vi "Configure Data Logger.vi"(0 "VISA resource name":refnum<visa-resource-name>, 1 "Data Logging (0: Current)":i32(ring) items=["Current", "Voltage"], 5 "Channel (1)":string="1", 7 "Sample Duration (1 sec)":dbl=1.0, 9 "Sample Interval (0.2 sec)":dbl=0.2, 11 "error in (no error)":errorcluster, 12 "Enable Data Logging (T: Enable)":bool=TRUE, 13 "Enable Extremum (T: Enable)":bool=TRUE) -> (4 "VISA resource name out":refnum<visa-resource-name>, 15 "error out":errorcluster)   [LabVIEW 2020, in "Keysight E36300 Series.lvlib"]
doc: "Configures the data logging.\n\n<b>Note: </b>\nThis VI is only available on the E36312A and E36313A models."
uses:
  Keysight E36300 Series.lvlib
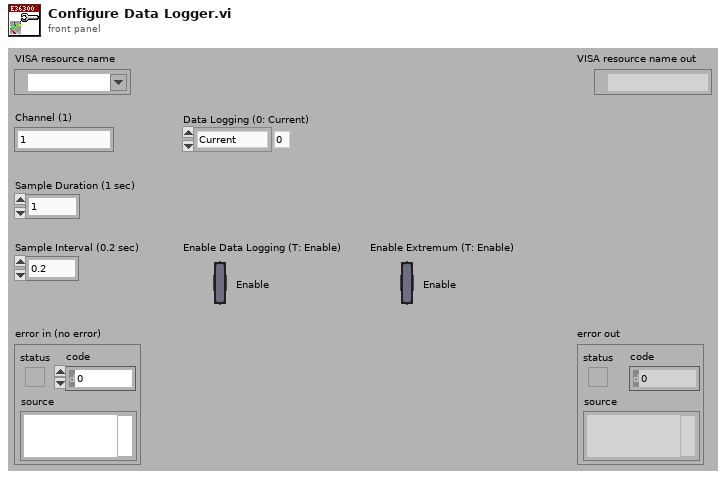
[diagram p1: front panel]
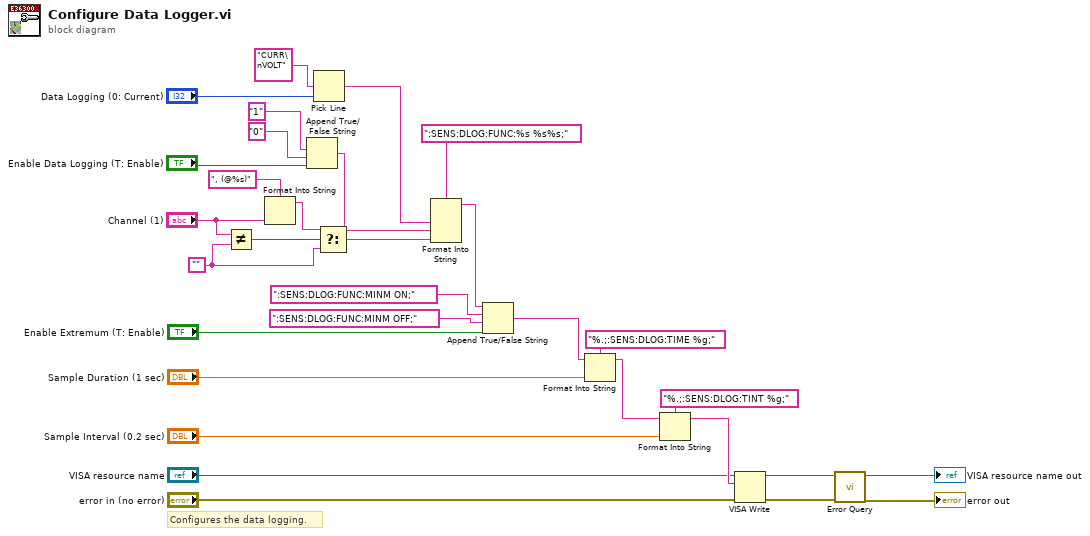
[diagram p0: block diagram]
diagram:
  w3 = ""
  # "Configures the data logging."
  n1 = Not Equal?(x="Channel (1)", y=w3) -> (x != y?=w1:bool)
  n2 = Format Into String(format string=", (@%s)", "Channel (1)") -> (resulting string=w5:string)  [unwired: 2 in, 1 out]
  n3 = Append True/False String(1:"Enable Data Logging (T: Enable)", 2:"0", 3:"1") -> (0:w24:string)  [unwired: 1 in]
  n4 = Pick Line(multi-line string="CURR\nVOLT", line index="Data Logging (0: Current)") -> (output string=w25:string)  [unwired: 1 in]
  n5 = Select(t=w5, s=w1, f=w3) -> (s? t:f=w4:string)
  n6 = Format Into String(format string=":SENS:DLOG:FUNC:%s %s%s;", w25, w24, w4) -> (resulting string=w23:string)  [unwired: 2 in, 1 out]
  n7 = Append True/False String(1:"Enable Extremum (T: Enable)", 2:":SENS:DLOG:FUNC:MINM OFF;", 3:":SENS:DLOG:FUNC:MINM ON;", 4:w23) -> (0:w6:string)
  n8 = Format Into String(format string="%.;:SENS:DLOG:TIME %g;", initial string=w6, "Sample Duration (1 sec)") -> (resulting string=w17:string)  [unwired: 1 in, 1 out]
  n9 = Format Into String(format string="%.;:SENS:DLOG:TINT %g;", initial string=w17, "Sample Interval (0.2 sec)") -> (resulting string=w14:string)  [unwired: 1 in, 1 out]
  n10 = VISA Write(VISA resource name="VISA resource name", write buffer=w14, error in (no error)="error in (no error)") -> (VISA resource name out=w11:refnum<visa-resource-name>, error out=w10:errorcluster)  [unwired: 1 out]
  n11 = call "Error Query.vi"("error in (no error)"=w10, "VISA resource name"=w11) -> ("error out"=→"error out":errorcluster, "VISA resource name out"=→"VISA resource name out":refnum<visa-resource-name>)  [unwired: 6 in, 2 out]
